vi "UpdateModeID.vi"(10 "Mode IDs":string[](array[string]), 11 "Array in":T1[](array[typedef])) -> (3 "Array out":T1[](array[typedef]))   [LabVIEW 2018]
uses:
  Controls/Holo Setting.ctl
  Controls/Buttons/Running Button.ctl
  Controls/Zernike Polynominals.ctl
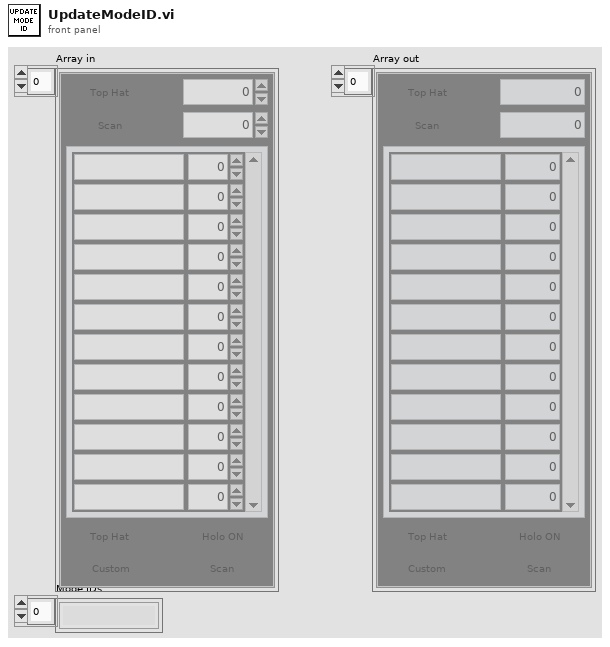
[diagram p1: front panel]
types:
  T1 = typedef "Holo Setting.ctl" = cluster{"Holo On":T2, "Scan":T2, "X":i16, "Y":i16, "Zernike Polynominals":T3, "Top Hat":T2, "Vortex":T2, "Clockwise":T2, "Custom":T2}
  T2 = typedef "Running Button.ctl" = bool
  T3 = typedef "Zernike Polynominals.ctl" = cluster{"Aberration Name":string, "Numeric":dbl}[]
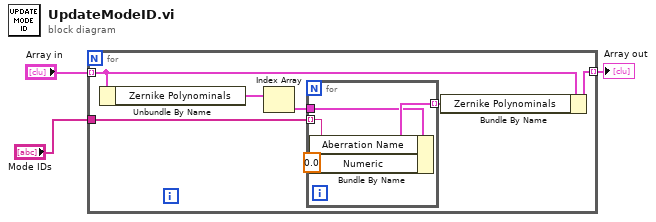
[diagram p0: block diagram]
diagram:
  n1 = for {
    tunnel: "Array in" -> [w8] mode=indexing
    tunnel: "Mode IDs" -> [w9]
    tunnel: [w6] -> w2 mode=indexing
    n2 = Unbundle By Name(w8) -> ("Zernike Polynominals"=w5:T3)
    n3 = Index Array(array=w5) -> (element=w4:cluster{"Aberration Name":string, "Numeric":dbl})  [unwired: 1 in]
    n4 = for {
      tunnel: w9 -> [w13] mode=indexing
      tunnel: [w12] -> w7 mode=indexing
      tunnel: w4 -> [w11]
      n5 = Bundle By Name(cluster=w11, "Aberration Name"=w13, "Numeric"=0.0 ("Amplititute")) -> (w12:cluster{"Aberration Name":string, "Numeric":dbl})
    }
    n6 = Bundle By Name(cluster=w8, "Zernike Polynominals"=w7) -> (w6:T1)
  }
  "Array out" <- w2
